vi "FTW-Messenger-Actor-RequestShutdown.vi"(0 "Messenger":refnum<class "FTW-Messenger-Actor.lvclass">, 5 "Shutdown Payload Message":refnum<class "FTW-Message.lvclass">, 11 "error in":errorcluster) -> (4 "Messenger out":refnum<class "FTW-Messenger-Actor.lvclass">, 15 "error out":errorcluster)   [LabVIEW 2014, in "FTW-Messenger-Actor.lvclass"]
uses:
  FTW-Messenger-Actor.lvclass
  Message/FTW-Message.lvclass
panel:
  # "Inputs"
  # "Outputs"
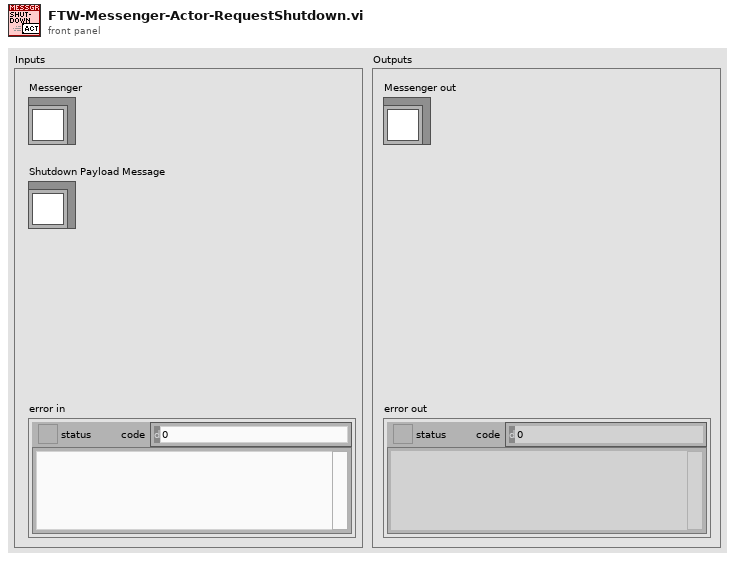
[diagram p1: front panel]
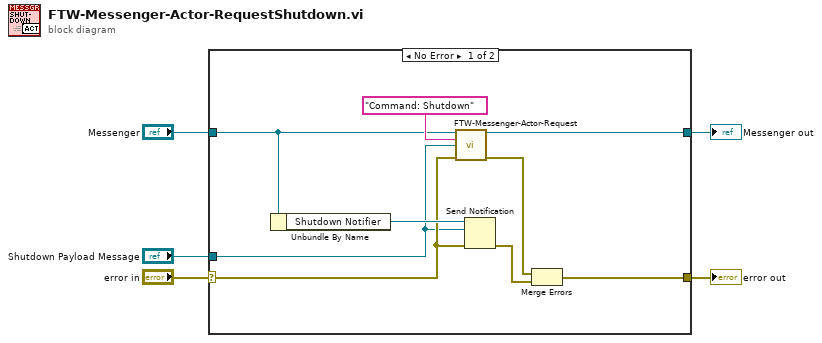
[diagram p0: block diagram]
diagram:
  n1 = case shown="No Error" "error in" {
    selector: "error in" -> [w10 w16]
    tunnel: [w6 w16] -> w4
    tunnel: [w14 w15] -> w5
    tunnel: "Messenger" -> [w12 w15]
    tunnel: "Shutdown Payload Message" -> [w9 _]
    frame No Error {
      n2 = Unbundle By Name(w12) -> ("Shutdown Notifier"=w11:refnum<notifier>)
      n3 = call-dynamic "FTW-Messenger-Actor-Request.vi"("Messenger"=w12, "Parameter"="Command: Shutdown", "Payload"=w9, "error in"=w10) -> ("Messenger out"=w14:refnum<class "FTW-Messenger-Actor.lvclass">, "error out"=w7:errorcluster)  [unwired: 10 in]
      n4 = Send Notification(notification=w9, notifier=w11, error in (no error)=w10) -> (error out=w8:errorcluster)  [unwired: 1 out]
      n5 = Merge Errors(w7, w8) -> (w6:errorcluster)
    }
    frame Error {
    }
  }
  "Messenger out" <- w5
  "error out" <- w4
